vi "LV86_Morph_ExternalEdge.vi"(2 "Connectivity":enum16{"4", "6", "8"}(ring), 3 "Image in":T1 {"Dialogs" format="%.0b"}) -> (1 "Image out":T1 {"Dialogs" format="%.0b"})   [LabVIEW 2024]
doc: "This VI performs an external egde detection on the input image. The result is an image containing only the external edges of the features in the original image."
uses:
  <userlib>/ImageProcessing/QTLIB_2595_LV86/QT_Image.ctl
panel:
  out "External Edge":picture caption="new picture"
  out "Initial Image":picture caption="new picture"
  # "Initial Image"
  # "This VI performs an external egde detection on the \ninput image.  The result is an image containing only \nthe external edges of the features in the original image."
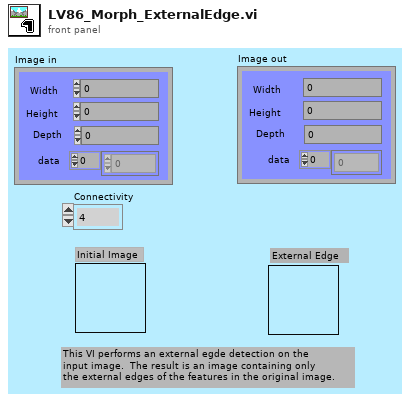
[diagram p1: front panel]
types:
  T1 = typedef "QT_Image.ctl" = cluster{"Width":i32, "Height":i32, "Depth":i32, "data":u8[], "Compressed data":u8[], "Color table":u32[], "Duration":i32, "Options":i32, "Timestamp":i32, "ID":i32, "Reserved":i32, "Dialogs":u32}
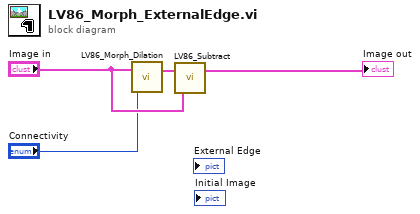
[diagram p0: block diagram]
diagram:
  n1 = call <userlib>:"LV86_Morph_Dilation.vi"("Connectivity"="Connectivity", "Image in"="Image in") -> ("Image out"=w2:T1)  [unwired: 1 out]
  n2 = call <userlib>:"LV86_Subtract.vi"("Image 2"="Image in", "Image"=w2) -> ("Image Out"=→"Image out":T1)  [unwired: 1 in]
